vi "应变数据转化.vi"(1 "应变数据转换配置":T1={"电桥"="全桥", "ADC精度"=0.0, "增益倍数"=0.0, "参考电压"=0.0, "应变片灵敏度"=0.0}, 2 "原始数据入":string) -> (0 "应变":dbl format="%#_6p ε")   [LabVIEW 2019]
panel:
  # "IN"
  # "OUT"
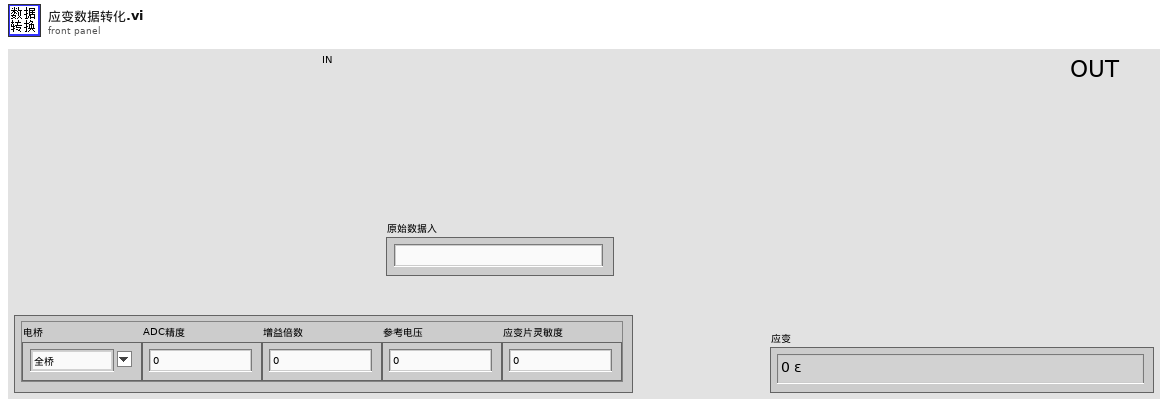
[diagram p1: front panel]
types:
  T1 = cluster{"电桥":string, "ADC精度":dbl, "增益倍数":dbl, "参考电压":dbl, "应变片灵敏度":dbl}
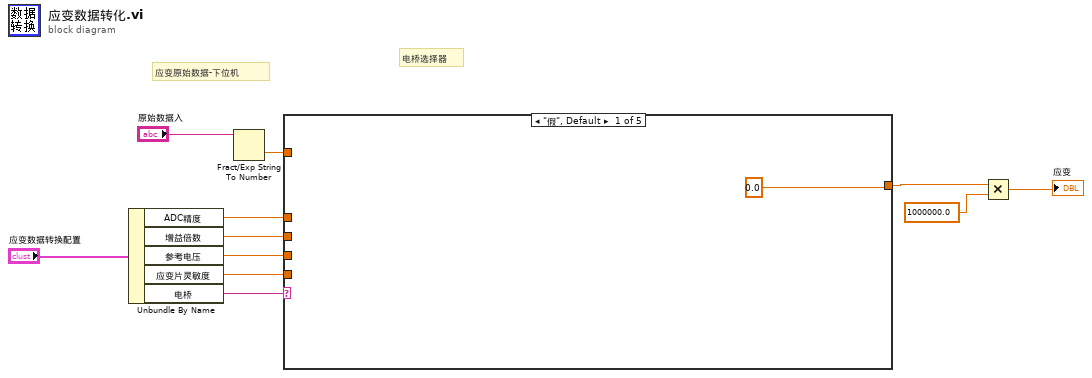
[diagram p0: block diagram]
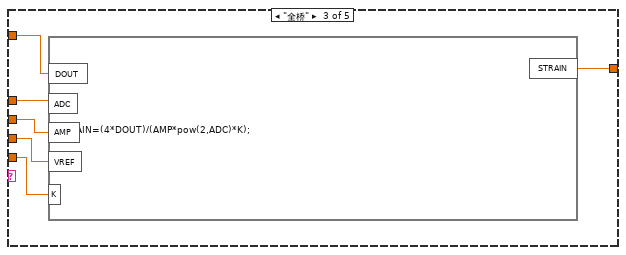
[diagram p3: hidden frame]
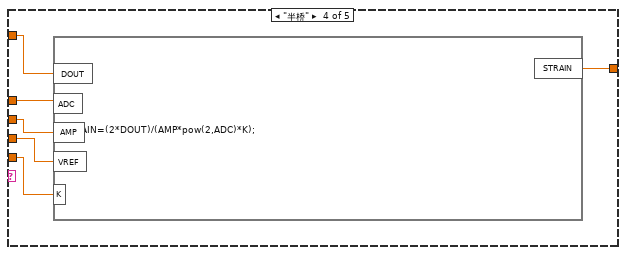
[diagram p4: hidden frame]
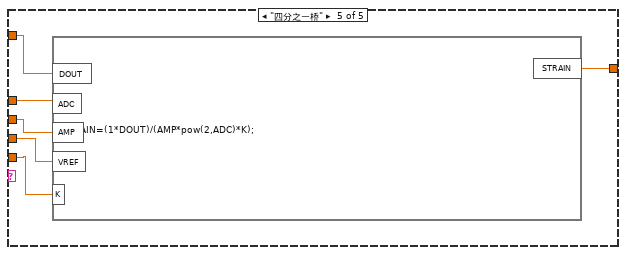
[diagram p5: hidden frame]
diagram:
  # "应变原始数据-下位机"
  # "电桥选择器"
  n1 = Unbundle By Name("应变数据转换配置") -> ("ADC精度"=w5:dbl, "增益倍数"=w6:dbl, "参考电压"=w7:dbl, "应变片灵敏度"=w8:dbl, "电桥"=w9:string)
  n2 = Fract/Exp String To Number(string="原始数据入") -> (number=w10:dbl)  [unwired: 3 in, 1 out]
  n3 = case shown="\"假\", Default" w9 {
    tunnel: w10 -> [_ w13 w19 w20 w30]
    tunnel: w8 -> [_ _ w18 w24 w26]
    tunnel: w7 -> [_ _ w17 w23 w27]
    tunnel: w6 -> [_ _ w16 w22 w28]
    tunnel: w5 -> [_ _ w15 w21 w29]
    tunnel: [0.0 ("strain") w13 w14 w25 w31] -> w3
    frame "假", Default {
    }
    frame "不使用" {
    }
    frame "全桥" {
      n4 = formula code="STRAIN=(4*DOUT)/(AMP*pow(2,ADC)*K);"("DOUT"=w19, "AMP"=w16, "ADC"=w15, "VREF"=w17, "K"=w18) -> ("STRAIN"=w14:dbl)
    }
    frame "半桥" {
      n5 = formula code="STRAIN=(2*DOUT)/(AMP*pow(2,ADC)*K);"("DOUT"=w20, "AMP"=w22, "ADC"=w21, "VREF"=w23, "K"=w24) -> ("STRAIN"=w25:dbl)
    }
    frame "四分之一桥" {
      n6 = formula code="STRAIN=(1*DOUT)/(AMP*pow(2,ADC)*K);"("DOUT"=w30, "AMP"=w28, "ADC"=w29, "VREF"=w27, "K"=w26) -> ("STRAIN"=w31:dbl)
    }
  }
  n7 = Multiply(x=w3, y=1000000.0) -> (x*y=→"应变":dbl)
